vi "xeva-abortAcquisition.vi"(3 "error in (no error)":errorcluster, 5 "Cam Ref":T1) -> (0 "error out":errorcluster, 1 "aborted":bool, 2 "Cam Ref Out":T1)   [LabVIEW 2017]
uses:
  <vilib>/Xenics Infrared Solutions/Xeneth LabVIEW API/VIs/Controls/Camara.ctl
  <vilib>/Xenics Infrared Solutions/Xeneth LabVIEW API/Xeneth.lvlib
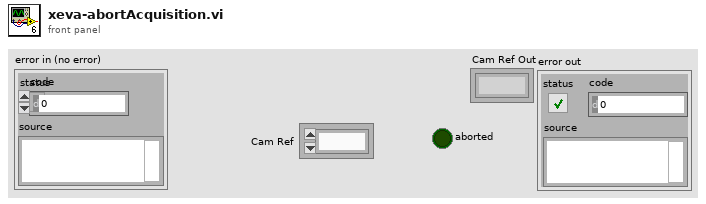
[diagram p1: front panel]
types:
  T1 = typedef "Xeneth.lvlib/Camara.ctl" = refnum<k1>
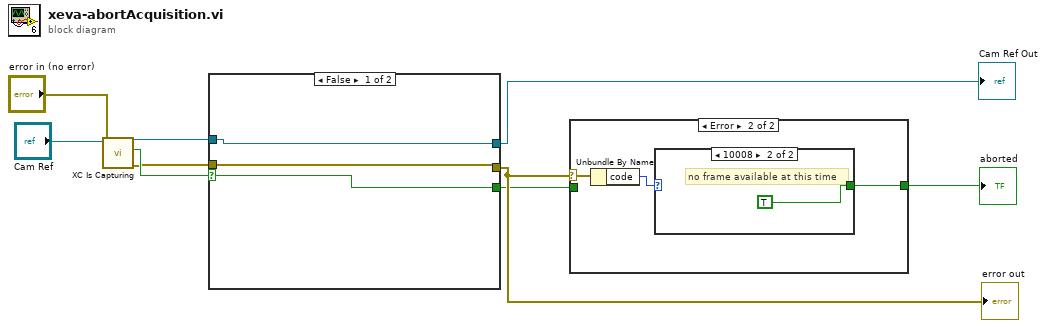
[diagram p0: block diagram]
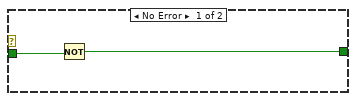
[diagram p2: hidden frame]
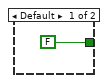
[diagram p3: hidden frame]
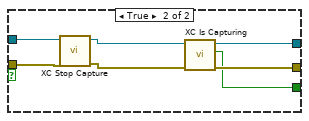
[diagram p4: hidden frame]
diagram:
  n1 = call <vilib>:"XC Is Capturing.vi"("error in (no error)"="error in (no error)", "Cam Ref"="Cam Ref") -> ("error out"=w7:errorcluster, "IsCapturing"=w8:bool, "Cam Ref Out"=w6:T1)  [unwired: 7 in]
  n2 = case shown="False" w8 {
    selector: w8 -> [w12 _]
    tunnel: w7 -> [w11 w19]
    tunnel: w6 -> [w10 w18]
    tunnel: [w11 w16] -> w5
    tunnel: [w12 w14] -> w4
    tunnel: [w10 w13] -> w3
    frame False {
    }
    frame True {
      n3 = call <vilib>:"XC Stop Capture.vi"("error in (no error)"=w19, "Cam Ref"=w18) -> ("error out"=w17:errorcluster, "Cam Ref Out"=w15:T1)  [unwired: 8 in]
      n4 = call <vilib>:"XC Is Capturing.vi"("error in (no error)"=w17, "Cam Ref"=w15) -> ("error out"=w16:errorcluster, "IsCapturing"=w14:bool, "Cam Ref Out"=w13:T1)  [unwired: 7 in]
    }
  }
  "Cam Ref Out" <- w3
  "error out" <- w5
  n5 = case shown="Error" w5 {
    selector: w5 -> [_ w24]
    tunnel: w4 -> [w21 _]
    tunnel: [w20 w22] -> w2
    frame No Error {
      n6 = Not(x=w21) -> (.not. x?=w20:bool)
    }
    frame Error {
      n7 = Unbundle By Name(w24) -> ("code"=w23:i32)
      n8 = case shown="10008" w23 {
        tunnel: [FALSE TRUE] -> w22
        frame Default {
        }
        frame 10008 {
          # "no frame available at this time"
        }
      }
    }
  }
  "aborted" <- w2
